vi "Interface Read N End Time.vi"(7 "count (1)":i32=1, 8 "error in (no error)":errorcluster, 11 "Dispatcher Interface in":refnum<class "Dispatcher Interface.lvclass">) -> (0 "error out":errorcluster, 1 "arg1":u64, 2 "us count":u32, 3 "Dispatcher Interface out":refnum<class "Dispatcher Interface.lvclass">)   [LabVIEW 2017]
uses:
  Classes/Interfaces/Dispatcher/Dispatcher Interface.lvclass
  C:/Git/DSF/Data Sharing Framework/Source/Core/Engine/Classes/Interfaces/Interface/Interface.lvclass
  Classes/Interfaces/Interface/Interface.lvclass/Interface.ctl
  Classes/Debug/FIFO Flags/FIFO Flags.lvclass/FIFO Flags.ctl
  Classes/Interfaces/Dispatcher/Read Dispatcher Command.vi
  Classes/Interfaces/Interface/Read Command.vi
  Classes/Interfaces/Interface/Get Command FIFO.vi
  Classes/Interfaces/Interface/Get Debug Flags.vi
  Classes/Interfaces/Interface/Read RT FIFO(16B).vi
  Classes/Debug/FIFO Flags/Get Infinite Timeouts.vi
  Classes/Interfaces/Interface/Errors.vi
  Classes/Interfaces/Interface/Command Timeout.vi
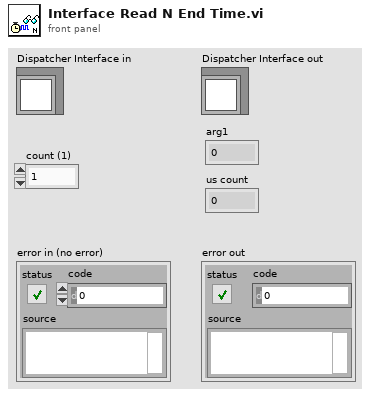
[diagram p1: front panel]
types:
  T1 = typedef "DSF Core.lvlib/Dispatcher Interface.lvclass/Command Data.ctl" = cluster{"Command":T2, "Parameters":T3}
  T2 = typedef "DSF Core.lvlib/Dispatcher Interface.lvclass/Command.ctl" = enum8{"Rx", "Tx", "Shutdown"}
  T3 = typedef "DSF Core.lvlib/Dispatcher Interface.lvclass/Parameters.ctl" = cluster{"arg1":u64, "arg2":u64}
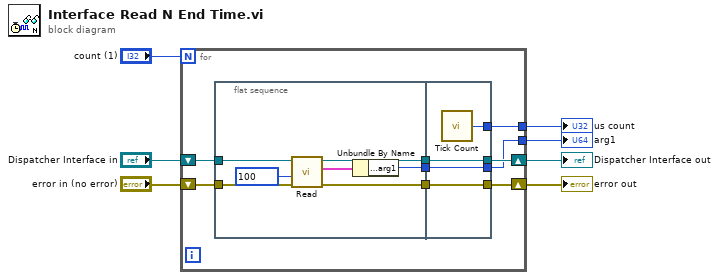
[diagram p0: block diagram]
diagram:
  n1 = for {
    N: "count (1)" -> [_]
    shift-right: [w14] -> w4
    shift-left: "Dispatcher Interface in" -> [w15]
    shift-right: [w13] -> w3
    shift-left: "error in (no error)" -> [w16]
    tunnel: [w10] -> w1
    tunnel: [w8] -> w2
    n2 = flat-sequence {
      tunnel: w16 -> [w23]
      tunnel: w15 -> [w22]
      tunnel: [w21] -> w12
      tunnel: [w20] -> w11
      tunnel: [w17] -> w9
      tunnel: [w26] -> w13
      tunnel: [w27] -> w14
      tunnel: w12 -> [w27]
      tunnel: w11 -> [w26]
      tunnel: [w25] -> w10
      tunnel: w9 -> [w24]
      tunnel: [w24] -> w8
      frame #0 {
        n3 = call-poly "Read.vi"("error in (no error)"=w23, "timeout in ms (0)"=100, "Dispatcher Interface in"=w22) -> ("error out"=w20:errorcluster, "command"=w18:T1, "Dispatcher Interface out"=w21:refnum<class "Dispatcher Interface.lvclass">)  [unwired: 4 in, 2 out]
        n4 = Unbundle By Name(w18) -> ("Parameters.arg1"=w17:u64)
      }
      frame #1 {
        n5 = call "Tick Count"() -> ("Tick Count(uSec)"=w25:u32)
      }
    }
  }
  "Dispatcher Interface out" <- w4
  "error out" <- w3
  "arg1" <- w2
  "us count" <- w1
